vi "Read Room Number.vi"(8 "error in (no error)":errorcluster, 11 "Room in":refnum<class "Room.lvclass">) -> (0 "error out":errorcluster, 2 "Room Number":u8, 3 "Room out":refnum<class "Room.lvclass">)   [LabVIEW 2015, in "Room.lvclass"]
uses:
  Room.lvclass
  Room.lvclass/Room.ctl
  Flags/Flags.lvclass/Flags.ctl
  Flags/Flags.lvclass
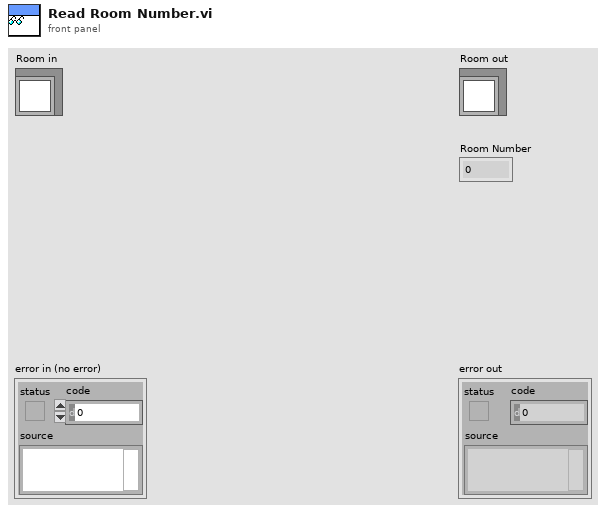
[diagram p1: front panel]
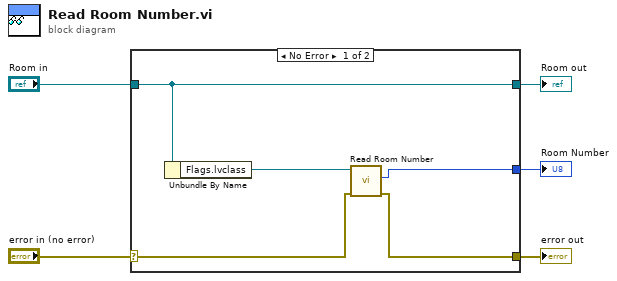
[diagram p0: block diagram]
diagram:
  n1 = case shown="No Error" "error in (no error)" {
    selector: "error in (no error)" -> [w7 w11]
    tunnel: [w6 w11] -> w4
    tunnel: [w10 w12] -> w2
    tunnel: "Room in" -> [w10 w12]
    tunnel: [w8 _] -> w1
    frame No Error {
      n2 = Unbundle By Name(w10) -> ("Flags.lvclass"=w9:refnum<class "Flags.lvclass">)
      n3 = call "Read Room Number.vi"("error in (no error)"=w7, "Flags in"=w9) -> ("error out"=w6:errorcluster, "Room Number"=w8:u32)  [unwired: 7 in, 1 out]
    }
    frame Error {
    }
  }
  "error out" <- w4
  "Room out" <- w2
  "Room Number" <- w1
